vi "update config.vi"(8 "error in (no error)":errorcluster, 10 "user configurations":T2={"vst_device"=["VST_1", "VST_2"], "RF gain "=10.0, "buffer size"=524288, "center frequency (Hz) "=1000000000.0, "P2P sample rate"=200000000.0, "mode"=enum."5785 - 2*180MHz", "devicess"=["IF_transiver_0", "IF_transiver_1", "IF_transiver_2"], "file paths"=[path "C:/Users/PXIe8108_Demo/Documents/CHAIM DATA/chaim/5785_sync_for_elbit/data/pdw_test_file.tdms", path "C:/Users/PXIe8108_Demo/Documents/CHAIM DATA/chaim/5785_sync_for_elbit/data/pdw_test_file_1.tdms", path "C:/Users/PXIe8108_Demo/Documents/CHAIM DATA/chaim/5785_sync_for_elbit/data/pdw_test_file_2.tdms", path "C:/Users/PXIe8108_Demo/Documents/CHAIM DATA/chaim/5785_sync_for_elbit/data/pdw_test_file_3.tdms", path "C:/Users/PXIe8108_Demo/Documents/CHAIM DATA/chaim/5785_sync_for_elbit/data/pdw_test_file_4.tdms"], "gen for df"=FALSE}, 11 "5785_2_x_200MHz in":refnum<class "5785_2_x_200MHz.lvclass">) -> (0 "error out":errorcluster, 1 "min frequency":dbl, 2 "max frequency":dbl, 3 "5785_2_x_200MHz out":refnum<class "5785_2_x_200MHz.lvclass">)   [LabVIEW 2021, in "5785_2_x_200MHz.lvclass"]
uses:
  <vilib>/userdefined/High Color/nirio_resource_hc.ctl
  5785_2_x_200MHz.lvclass
  5785_2_x_200MHz.lvclass/5785_2_x_200MHz.ctl
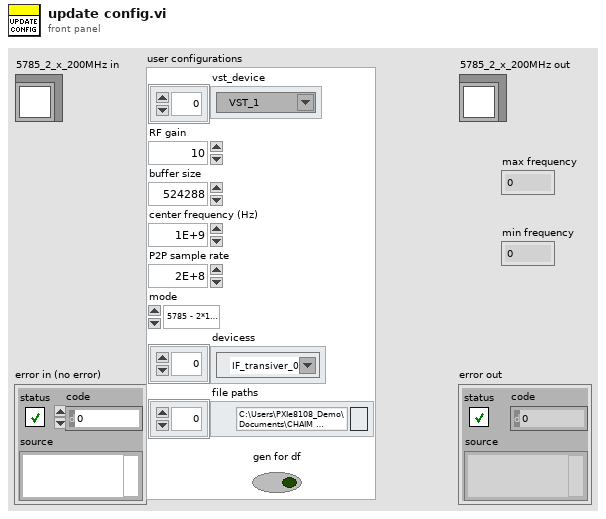
[diagram p1: front panel]
types:
  T1 = typedef "nirio_resource_hc.ctl" = tag
  T2 = cluster{"vst_device":refnum<k15>[], "RF gain ":dbl, "buffer size":u32, "center frequency (Hz) ":dbl, "P2P sample rate":dbl, "mode":enum16{"USRP - 180MHz", "5785 - 2*180MHz", "5785 - 3.2GHz", "P2P - VST"}, "devicess":T1[], "file paths":path[], "gen for df":bool}
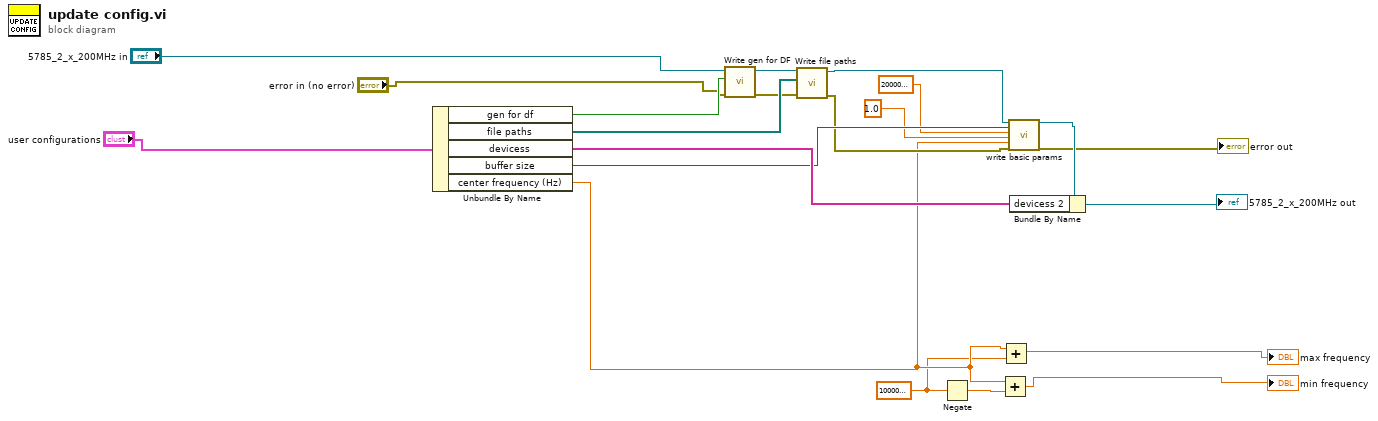
[diagram p0: block diagram]
diagram:
  w1 = 100000000.0 ("Fs  FPGA")
  n1 = Unbundle By Name("user configurations") -> ("gen for df"=w12:bool, "file paths"=w15:path[], "devicess"=w21:T1[], "buffer size"=w19:u32, "center frequency (Hz)"=w2:dbl)
  n2 = call-dynamic "Write gen for DF.vi"("error in (no error)"="error in (no error)", "gen for DF"=w12, "device_type in"="5785_2_x_200MHz in") -> ("error out"=w11:errorcluster, "device_type out"=w13:refnum<class "5785_2_x_200MHz.lvclass">)  [unwired: 7 in]
  n3 = call-dynamic "Write file paths.vi"("error in (no error)"=w11, "file paths"=w15, "device_type in"=w13) -> ("error out"=w10:errorcluster, "device_type out"=w14:refnum<class "5785_2_x_200MHz.lvclass">)  [unwired: 7 in]
  n4 = Negate(x=w1) -> (-x=w20:dbl)
  n5 = Add(x=w2, y=w20) -> (x+y=→"min frequency":dbl)
  n6 = Add(x=w2, y=w1) -> (x+y=→"max frequency":dbl)
  n7 = call-dynamic "write basic params.vi"("device_type in"=w14, "buffer size"=w19, "Fs  FPGA"=200000000.0, "SPC"=1.0 ("Fs  FPGA"), "center frequency (Hz)"=w2, "error in (no error)"=w10) -> ("device_type out"=w16:refnum<class "5785_2_x_200MHz.lvclass">, "error out"=→"error out":errorcluster)  [unwired: 12 in]
  n8 = Bundle By Name(cluster=w16, "devicess 2"=w21) -> (→"5785_2_x_200MHz out":refnum<class "5785_2_x_200MHz.lvclass">)
